vi "SS2 Live_Settings Window.vi"() -> ()   [LabVIEW 2019]
uses:
  SS2 DAQ Parameters 2.ctl
  SS2 Gate Definition.ctl
  SS2 Live_File Information.ctl
  SS2 Live_Gate Characteristics.ctl
  SS2 Live_Image ROI Information.ctl
  Phasor/Image Binning Options.ctl
  SS2 Live_Settings Event.ctl
  SS2 Live_Settings Window Messages.ctl
  SS2 Live_Settings Q Action.ctl
  SS2 Live_Gate Configuration Action.ctl
  SS2 Live_Settings Q Element.ctl
  SS2 Gate Configuration.ctl
  SS2 Live_Globals.vi
  Variant/Variant to Data/Variant to Data.lvlib
panel:
  in  "Tab Control":T1(tab)
  in  "Bitfile Version":string
  in  "Bitfile Path":path
  in  "Buffer Size (# Gates)":u32=1 min=1
  out "Gate Characteristics":T2
  in  "Preset Configuration":u16(ring) items=["User-defined configuration", "Gate Configuration 1", "Gate Configuration 2", "Gate Configuration 3", "Gate Configuration 4", "Gate Configuration 5", "Gate Configuration 6", "Gate Configuration 7"]
  in  "SS2 DAQ Parameters":T3={"10 bits"=FALSE, "# Exposure Sequences"=1, "# 1-bit Frame per Gate"=255, "Gate Shift"=0, "# Gates per Set"=1, "# Sets"=1, "Laser Period"=0.0, "Gate Offset"=0, "Auto-adjust Gate Offset"=FALSE, "Gate Definition"={"gs_psincdec_0"=0, "gs_psincdec_1"=0, "gs_psincdec_2"=0, "gs_psincdec_3"=0, "gs_no_shift_adj_1"=0, "gs_no_shift_adj_2"=0, "gs_no_shift_adj_3"=0}} {"Laser Period" min=0.0; "# 1-bit Frame per Gate" min=255 max=255; "Gate Definition"."gs_psincdec_3" max=1; "Gate Definition"."gs_psincdec_2" max=1; "Gate Definition"."gs_psincdec_1" max=1; "Gate Definition"."gs_psincdec_0" max=1; "# Sets" min=1; "# Gates per Set" min=1}
  in  "Image Binning Options":T5={"Use Image Binning"=FALSE, "X Bin"=1, "Y Bin"=1} {"Y Bin" min=1; "X Bin" min=1}
  in  "Image ROI Information":T6
  in  "# Datasets in Series":i32=1 min=1
  in  "File Information":T7
  in  "Histogram Bins Number":i32=256 min=1 step=1
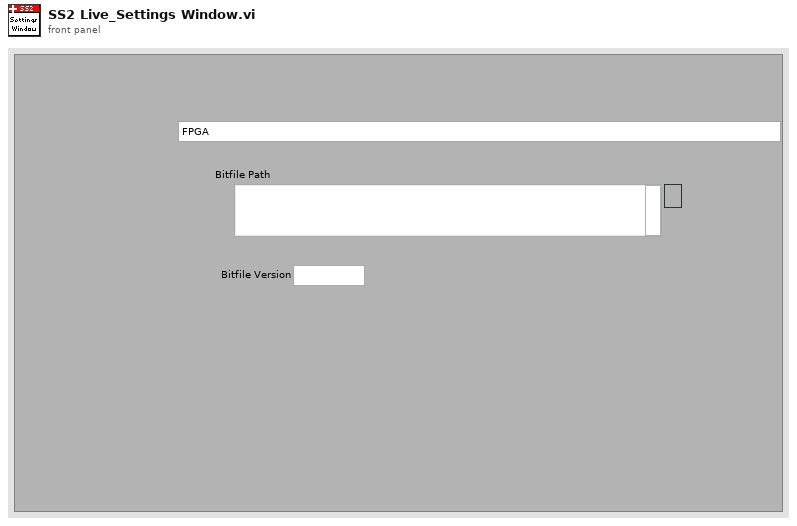
[diagram p1: front panel]
types:
  T1 = enum32{"FPGA", "Acquisition Parameters", "Image Parameters", "File Information", "UI Parameters"}
  T2 = typedef "SS2 Live_Gate Characteristics.ctl" = cluster{"Predicted Gate Width":dbl[unit], "Gate Image Duration":dbl[unit], "Gate Image Exposure":dbl[unit], "Gate Shift":dbl[unit], "Gate Images Span":dbl[unit]}
  T3 = typedef "SS2 DAQ Parameters 2.ctl" = cluster{"10 bits":bool, "# Exposure Sequences":u32, "# 1-bit Frame per Gate":u32, "Gate Shift":u32, "# Gates per Set":u32, "# Sets":u32, "Laser Period":dbl[unit], "Gate Offset":u32, "Auto-adjust Gate Offset":bool, "Gate Definition":T4}
  T4 = typedef "SS2 Gate Definition.ctl" = cluster{"gs_psincdec_0":u32, "gs_psincdec_1":u32, "gs_psincdec_2":u32, "gs_psincdec_3":u32, "gs_no_shift_adj_1":u32, "gs_no_shift_adj_2":u32, "gs_no_shift_adj_3":u32}
  T5 = typedef "Image Binning Options.ctl" = cluster{"Use Image Binning":bool, "X Bin":i32, "Y Bin":i32}
  T6 = typedef "SS2 Live_Image ROI Information.ctl" = cluster{"Save ROI Only":bool, "Left":u16, "Top":u16, "Right":u16, "Bottom":u16, "Use Current ROI":bool}
  T7 = typedef "SS2 Live_File Information.ctl" = cluster{"File Folder":path, "File Name":string, "File Index":u32, "Author":string, "Sample":string, "Compression":bool}
  T8 = typedef "SS2 Live_Settings Q Action.ctl" = enum16{"Idle", "Store Current Configuration", "Rename Current Configuration", "Delete Current Configuration", "Update Image ROI Information", "Quit"}
  T9 = typedef "SS2 Live_Settings Event.ctl" = cluster{"Settings Message":T10, "Sender":string, "Control Label":string, "Data":variant}
  T10 = typedef "SS2 Live_Settings Window Messages.ctl" = enum16{"Idle", "Subscribe", "Unsubscribe", "Refresh Parameter", "Refresh All Parameters", "Quit"}
  T11 = typedef "SS2 Live_Gate Configuration Action.ctl" = enum16{"Get Gate Configuration Name", "Get Configuration by Name", "Add Gate Configuration", "Delete Gate Configuration", "Rename Gate Configuration"}
  T12 = typedef "SS2 Live_Settings Q Element.ctl" = cluster{"Action":T8, "Data":variant}
  T13 = typedef "SS2 Gate Configuration.ctl" = cluster{"Gate Configuration":string, "Gate Offset":u32, "Gate Definition":T4}
  T14 = enum32{"Invalid", "Standard", "Closed", "Hidden", "Minimized", "Maximized"}
  T15 = typedef "SS2 DAQ_Settings Window Messages.ctl" = enum16{"Idle", "Subscribe", "Unsubscribe", "Refresh Parameter", "Refresh All Parameters", "Quit"}
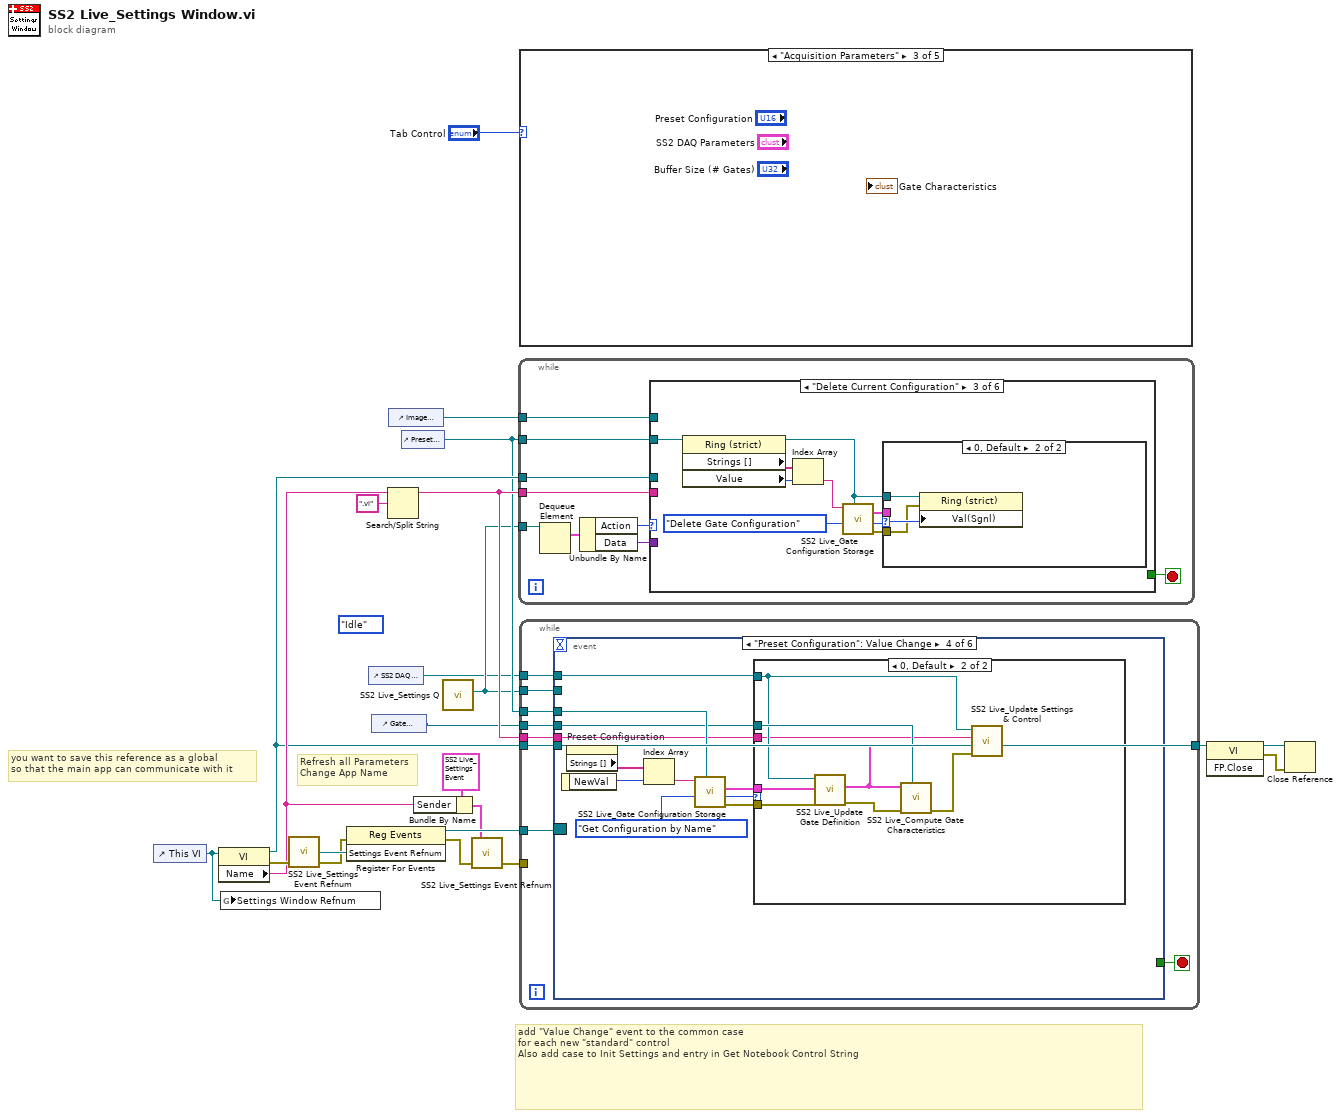
[diagram p0: block diagram]
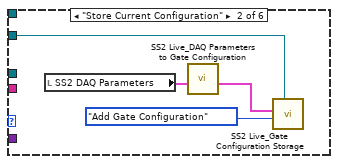
[diagram p3: hidden frame]
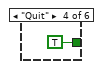
[diagram p5: hidden frame]
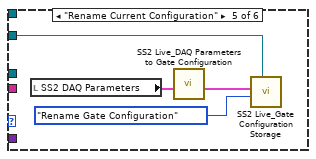
[diagram p6: hidden frame]
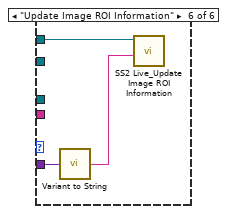
[diagram p7: hidden frame]
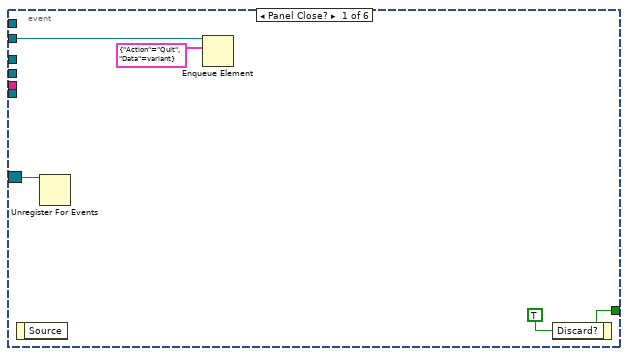
[diagram p8: hidden frame]
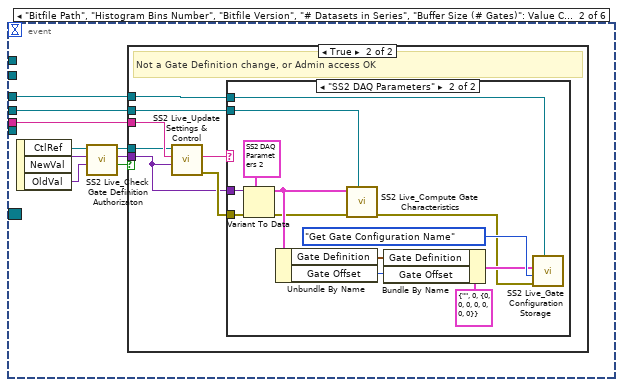
[diagram p9: hidden frame]
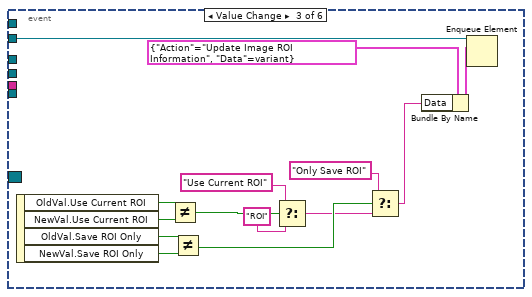
[diagram p12: hidden frame]
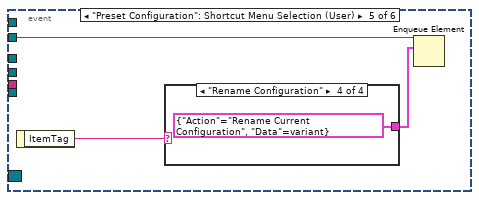
[diagram p14: hidden frame]
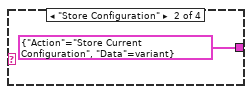
[diagram p16: hidden frame]
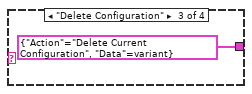
[diagram p17: hidden frame]
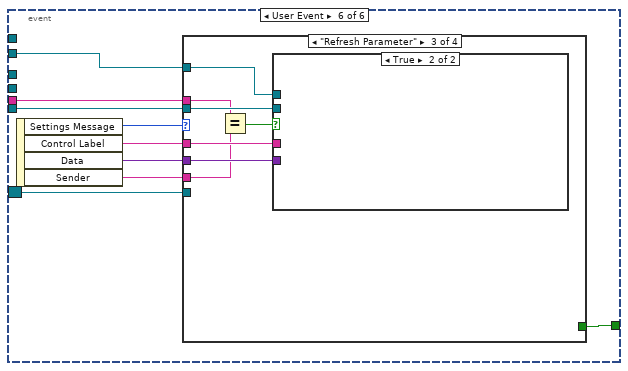
[diagram p18: hidden frame]
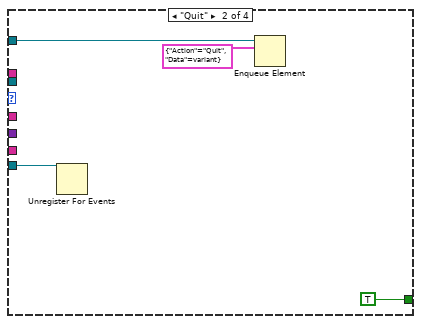
[diagram p20: hidden frame]
diagram:
  (unwired) SS2_Live_Settings_Q_Action."Idle" ("Action")
  # "you want to save this reference as a global\nso that the main app can communicate with it"
  # "add \"Value Change\" event to the common case\nfor each new \"standard\" control\nAlso add case to Init Settings and entry in Get Notebook Control String"
  # "Refresh all Parameters\nChange App Name"
  n1 = control-ref of="This VI"() -> (w6:refnum<vi>)
  n2 = property class="VI"(reference=w6) -> (reference out=w7:refnum<vi>, error out=w16:errorcluster, "Name"=w14:string)  [unwired: 1 in]
  n3 = global write "SS2 Live_Globals.vi" "Settings Window Refnum"(w6) -> ()
  n4 = call "SS2 Live_Settings Event Refnum.vi"("Error In"=w16) -> ("Settings Event Refnum"=w22:refnum<user-event>, "Error Out"=w21:errorcluster)  [unwired: 7 in]
  n5 = register-events(error in=w21, w22) -> (reference out=w19:refnum<event-registration>, error out=w18:errorcluster)  [unwired: 1 in]
  n6 = control-ref of="SS2 DAQ Parameters"() -> (w1:refnum<vi>)
  n7 = control-ref of="Gate Characteristics"() -> (w2:refnum<vi>)
  n8 = Search/Split String(string=w14, search string/char (-)=".vi") -> (substring before match=w9:string)  [unwired: 1 in, 2 out]
  n9 = control-ref of="Image Information"() -> (w4:refnum<vi>)
  n10 = control-ref of="Preset Configuration"() -> (w5:refnum<vi>)
  n11 = Bundle By Name(cluster=T9 {"Settings Message"=enum."Refresh All Parameters", "Sender"="Settings Window", "Control Label"="", "Data"=variant} ("Settings Event"), "Sender"=w14) -> (w15:T9)
  n12 = call "SS2 Live_Settings Q.vi"() -> ("Queue out"=w3:refnum<queue>)  [unwired: 10 in, 1 out]
  n13 = call "SS2 Live_Settings Event Refnum.vi"("Settings Event"=w15, "Error In"=w18) -> ("Error Out"=w12:errorcluster)  [unwired: 6 in, 1 out]
  n14 = while {
    tunnel: w3 -> [w31]
    tunnel: w9 -> [w26]
    tunnel: w7 -> [w25]
    tunnel: w5 -> [w24]
    tunnel: w4 -> [w23]
    stop <- w28 stop-if-true
    n15 = Dequeue Element(queue=w31) -> (element=w30:T12)  [unwired: 2 in, 3 out]
    n16 = Unbundle By Name(w30) -> ("Action"=w29:T8, "Data"=w27:variant)
    n17 = case shown="\"Delete Current Configuration\"" w29 {
      tunnel: [_ _ _ TRUE _ _] -> w28
      tunnel: w27 -> [_ _ _ _ _ w54]
      tunnel: w26 -> [_ _ _ _ _ _]
      tunnel: w25 -> [_ _ _ _ _ _]
      tunnel: w24 -> [_ w32 w43 _ w49 _]
      tunnel: w23 -> [_ _ _ _ _ w55]
      frame "Idle", Default {
      }
      frame "Store Current Configuration" {
        n18 = local read "SS2 DAQ Parameters"() -> (w34:T3)
        n19 = call "SS2 Live_DAQ Parameters to Gate Configuration.vi"("SS2 DAQ Parameters"=w34) -> ("Gate Configuration Definition out"=w33:T13)  [unwired: 10 in]
        n20 = call "SS2 Live_Gate Configuration Storage.vi"("Preset Configuration Refnum"=w32, "Action"=SS2_Live_Gate_Configuration_Action."Add Gate Configuration", "Gate Configuration Definition in"=w33) -> ()  [unwired: 3 in, 6 out]
      }
      frame "Delete Current Configuration" {
        n21 = property class="Ring (strict)"(reference=w43) -> (reference out=w37:refnum<vi>, "Strings []"=w42:string[], "Value"=w41:u16)  [unwired: 1 in, 1 out]
        n22 = Index Array(array=w42, index=w41) -> (element=w40:string)
        n23 = call "SS2 Live_Gate Configuration Storage.vi"("Preset Configuration Refnum"=w37, "Action"=SS2_Live_Gate_Configuration_Action."Delete Gate Configuration", "Gate Configuration Name in"=w40) -> ("Error Out"=w36:errorcluster, "Configuration ID"=w39:i32, "Gate Configuration Definition out"=w38:T13)  [unwired: 3 in, 3 out]
        n24 = case shown="0, Default" w39 {
          selector: w39 -> [_ w47]
          tunnel: w38 -> [_ _]
          tunnel: w37 -> [_ w46]
          tunnel: w36 -> [_ w45]
          frame -1 {
          }
          frame 0, Default {
            n25 = property class="Ring (strict)"(reference=w46, error in=w45, "Val(Sgnl)"=w47) -> ()  [unwired: 2 out]
          }
        }
      }
      frame "Quit" {
      }
      frame "Rename Current Configuration" {
        n26 = local read "SS2 DAQ Parameters"() -> (w51:T3)
        n27 = call "SS2 Live_DAQ Parameters to Gate Configuration.vi"("SS2 DAQ Parameters"=w51) -> ("Gate Configuration Definition out"=w50:T13)  [unwired: 10 in]
        n28 = call "SS2 Live_Gate Configuration Storage.vi"("Preset Configuration Refnum"=w49, "Action"=SS2_Live_Gate_Configuration_Action."Rename Gate Configuration", "Gate Configuration Definition in"=w50) -> ()  [unwired: 3 in, 6 out]
      }
      frame "Update Image ROI Information" {
        n29 = call "Variant to String.vi"("Variant"=w54) -> ("String"=w53:string)  [unwired: 8 in]
        n30 = call "SS2 Live_Update Image ROI Information.vi"("Element Changed"=w53, "Image Information Refnum"=w55) -> ()  [unwired: 8 in, 2 out]
      }
    }
  }
  n31 = case shown="\"Acquisition Parameters\"" "Tab Control" {
    frame "FPGA" {
    }
    frame "UI Parameters" {
    }
    frame "Acquisition Parameters" {
    }
    frame "Image Parameters" {
    }
    frame "File Information" {
    }
  }
  n32 = while {
    tunnel: w7 -> [w61]
    tunnel: [w61] -> w20
    tunnel: w19 -> [w62]
    tunnel: w9 -> [w60]
    tunnel: w12 -> [_]
    tunnel: w3 -> [w59]
    tunnel: w5 -> [w58]
    tunnel: w2 -> [w57]
    tunnel: w1 -> [w56]
    stop <- w63 stop-if-true
    n33 = event shown="[3] \"Preset Configuration\": Value Change" {
      selector: w62 -> [w66 _ _ _ _ w136]
      dyn-events: _ -> [_ _ _ _ _ _]
      timeout: _ -> [_ _ _ _ _ _]
      tunnel: [w67 _ _ _ _ w138] -> w63
      tunnel: w61 -> [_ _ _ _ _ w141]
      tunnel: w60 -> [_ w75 _ w111 _ w139]
      tunnel: w59 -> [w65 _ w110 _ w132 w137]
      tunnel: w58 -> [_ w73 _ w115 _ _]
      tunnel: w57 -> [_ w68 _ w114 _ _]
      tunnel: w56 -> [_ _ _ w113 _ _]
      event Panel Close? {
        w67 = TRUE ("Discard?")
        n34 = event-data() -> ()  [unwired: 1 in, 1 out]
        n35 = Unregister For Events(event registration refnum=w66) -> ()  [unwired: 1 in, 1 out]
        n36 = Enqueue Element(queue=w65, element=T12 {"Action"=enum."Quit", "Data"=variant}) -> ()  [unwired: 2 in, 3 out]
        n37 = event-data("Discard?"=w67) -> ()  [unwired: 1 in, 1 out]
      }
      event "Bitfile Path", "Histogram Bins Number", "Bitfile Version", "# Datasets in Series", "Buffer Size (# Gates)": Value Change {
        n38 = event-data() -> ("CtlRef"=w76:refnum<vi>, "NewVal"=w74:variant, "OldVal"=w70:variant)  [unwired: 1 in]
        n39 = call "SS2 Live_Check Gate Definition Authorizaton.vi"("OldVal"=w70, "NewVal"=w74, "Control Refnum"=w76) -> ("Change Accepted?"=w69:bool, "NewVal"=w71:variant, "Control Refnum"=w72:refnum<vi>)  [unwired: 5 in, 1 out]
        n40 = case shown="True" w69 {
          tunnel: w75 -> [_ w83]
          tunnel: w73 -> [_ w80]
          tunnel: w72 -> [_ w79]
          tunnel: w71 -> [_ w78]
          tunnel: w68 -> [_ w77]
          frame False {
            # "Not admin & Gate Definition change cancelled"
          }
          frame True {
            # "Not a Gate Definition change, or Admin access OK"
            n41 = call "SS2 Live_Update Settings & Control.vi"("Value"=w78, "Sender"=w83, "CtlRef"=w79) -> ("Error Out"=w81:errorcluster, "Control Label"=w82:string)  [unwired: 7 in]
            n42 = case shown="\"SS2 DAQ Parameters\"" w82 {
              tunnel: w78 -> [_ w96]
              tunnel: w81 -> [_ w95]
              tunnel: w80 -> [_ w88]
              tunnel: w77 -> [_ w84]
              frame "", Default {
              }
              frame "SS2 DAQ Parameters" {
                n43 = Variant To Data(error in=w95, type=T3 {"10 bits"=FALSE, "# Exposure Sequences"=0, "# 1-bit Frame per Gate"=255, "Gate Shift"=0, "# Gates per Set"=0, "# Sets"=1, "Laser Period"=0.0, "Gate Offset"=0, "Auto-adjust Gate Offset"=FALSE, "Gate Definition"={"gs_psincdec_0"=0, "gs_psincdec_1"=0, "gs_psincdec_2"=0, "gs_psincdec_3"=0, "gs_no_shift_adj_1"=0, "gs_no_shift_adj_2"=0, "gs_no_shift_adj_3"=0}} ("SS2 DAQ Parameters"), Variant=w96) -> (data=w87:T3, error out=w86:errorcluster)
                n44 = Unbundle By Name(w87) -> ("Gate Definition"=w90:T4, "Gate Offset"=w89:u32)
                n45 = call "SS2 Live_Compute Gate Characteristics.vi"("Gate Characteristics Refnum"=w84, "Error In"=w86, "SS2 DAQ Parameters"=w87) -> ("Error Out"=w85:errorcluster)  [unwired: 7 in, 1 out]
                n46 = Bundle By Name(cluster=T13 {"Gate Configuration"="", "Gate Offset"=0, "Gate Definition"={"gs_psincdec_0"=0, "gs_psincdec_1"=0, "gs_psincdec_2"=0, "gs_psincdec_3"=0, "gs_no_shift_adj_1"=0, "gs_no_shift_adj_2"=0, "gs_no_shift_adj_3"=0}} ("Gate Configuration Definition in"), "Gate Definition"=w90, "Gate Offset"=w89) -> (w91:T13)
                n47 = call "SS2 Live_Gate Configuration Storage.vi"("Preset Configuration Refnum"=w88, "Error In"=w85, "Action"=SS2_Live_Gate_Configuration_Action."Get Gate Configuration Name", "Gate Configuration Definition in"=w91) -> ()  [unwired: 2 in, 6 out]
              }
            }
          }
        }
      }
      event Value Change {
        n48 = event-data() -> ("OldVal.Use Current ROI"=w107:bool, "NewVal.Use Current ROI"=w106:bool, "OldVal.Save ROI Only"=w103:bool, "NewVal.Save ROI Only"=w102:bool)  [unwired: 1 in]
        n49 = Not Equal?(x=w107, y=w106) -> (x != y?=w105:bool)
        n50 = Not Equal?(x=w103, y=w102) -> (x != y?=w100:bool)
        n51 = Select(t="Use Current ROI" ("name (unnamed)"), s=w105, f="ROI" ("name (unnamed)")) -> (s? t:f=w99:string)
        n52 = Select(t="Only Save ROI" ("name (unnamed)"), s=w100, f=w99) -> (s? t:f=w97:string)
        n53 = Bundle By Name(cluster=T12 {"Action"=enum."Update Image ROI Information", "Data"=variant} ("element"), "Data"=w97) -> (w108:T12)
        n54 = Enqueue Element(queue=w110, element=w108) -> ()  [unwired: 2 in, 3 out]
      }
      event "Preset Configuration": Value Change {
        n55 = event-data() -> ("NewVal"=w120:u16)  [unwired: 1 in]
        n56 = property on="Preset Configuration" class="Ring (strict)"() -> ("Strings []"=w121:string[])  [unwired: 2 in, 2 out]
        n57 = Index Array(array=w121, index=w120) -> (element=w119:string)
        n58 = call "SS2 Live_Gate Configuration Storage.vi"("Preset Configuration Refnum"=w115, "Action"=SS2_Live_Gate_Configuration_Action."Get Configuration by Name", "Gate Configuration Name in"=w119) -> ("Error Out"=w112:errorcluster, "Configuration ID"=w117:i32, "Gate Configuration Definition out"=w118:T13)  [unwired: 3 in, 3 out]
        n59 = case shown="0, Default" w117 {
          tunnel: w118 -> [_ w128]
          tunnel: w114 -> [_ w129]
          tunnel: w113 -> [_ w124]
          tunnel: w112 -> [_ w127]
          tunnel: w111 -> [_ w123]
          frame -1 {
          }
          frame 0, Default {
            n60 = call "SS2 Live_Update Gate Definition.vi"("error in (no error)"=w127, "Gate Configuration Definition"=w128, "SS2 DAQ Parameters Refnum"=w124) -> ("error out"=w126:errorcluster, "SS2 DAQ Parameters"=w122:T3)  [unwired: 7 in]
            n61 = call "SS2 Live_Compute Gate Characteristics.vi"("Gate Characteristics Refnum"=w129, "Error In"=w126, "SS2 DAQ Parameters"=w122) -> ("Error Out"=w125:errorcluster)  [unwired: 7 in, 1 out]
            n62 = call "SS2 Live_Update Settings & Control.vi"("Error In"=w125, "Value"=w122, "Sender"=w123, "CtlRef"=w124) -> ()  [unwired: 6 in, 2 out]
          }
        }
      }
      event "Preset Configuration": Shortcut Menu Selection (User) {
        n63 = event-data() -> ("ItemTag"=w131:string)  [unwired: 1 in]
        n64 = case shown="\"Rename Configuration\"" w131 {
          tunnel: [_ T12 {"Action"=enum."Store Current Configuration", "Data"=variant} ("element") T12 {"Action"=enum."Delete Current Configuration", "Data"=variant} ("element") T12 {"Action"=enum."Rename Current Configuration", "Data"=variant} ("element")] -> w130
          frame "", Default {
          }
          frame "Store Configuration" {
          }
          frame "Delete Configuration" {
          }
          frame "Rename Configuration" {
          }
        }
        n65 = Enqueue Element(queue=w132, element=w130) -> ()  [unwired: 2 in, 3 out]
      }
      event User Event {
        n66 = event-data() -> ("Settings Message"=w144:T15, "Control Label"=w143:string, "Data"=w142:variant, "Sender"=w140:string)  [unwired: 1 in]
        n67 = case shown="\"Refresh Parameter\"" w144 {
          tunnel: w143 -> [_ _ w153 _]
          tunnel: w142 -> [_ _ w154 _]
          tunnel: w141 -> [_ _ w155 w174]
          tunnel: w140 -> [_ _ w152 w175]
          tunnel: w139 -> [_ _ w151 w176]
          tunnel: [_ TRUE ("Discard?") _ _] -> w138
          tunnel: w137 -> [_ w147 w149 _]
          tunnel: w136 -> [_ w145 _ _]
          frame "Idle", Default {
          }
          frame "Quit" {
            n68 = Unregister For Events(event registration refnum=w145) -> ()  [unwired: 1 in, 1 out]
            n69 = Enqueue Element(queue=w147, element=T12 {"Action"=enum."Quit", "Data"=variant}) -> ()  [unwired: 2 in, 3 out]
          }
          frame "Refresh Parameter" {
            n70 = Equal?(x=w152, y=w151) -> (x = y?=w150:bool)
            n71 = case shown="True" w150 {
              tunnel: w155 -> [w159 _]
              tunnel: w154 -> [w157 _]
              tunnel: w153 -> [w158 _]
              tunnel: w149 -> [w156 _]
              frame False {
                n72 = case shown="\"Image Information\"" w158 {
                  selector: w158 -> [_ w165]
                  tunnel: w159 -> [_ w166]
                  tunnel: w157 -> [_ w164]
                  tunnel: w156 -> [w163 _]
                  frame "Image Information" {
                    n73 = Bundle By Name(cluster=T12 {"Action"=enum."Update Image ROI Information", "Data"=variant} ("element"), "Data"="Use Current ROI") -> (w161:T12)
                    n74 = Enqueue Element(queue=w163, element=w161) -> ()  [unwired: 2 in, 3 out]
                  }
                  frame "", Default {
                    n75 = call "SS2 Live_Refresh Single Parameter.vi"("Data"=w164, "Control Label"=w165, "VI Ref in"=w166) -> ()  [unwired: 8 in, 1 out]
                  }
                }
              }
              frame True {
              }
            }
          }
          frame "Refresh All Parameters" {
            n76 = First Call?() -> (First Call?: T/F=w172:bool)
            n77 = Not(x=w172) -> (.not. x?=w171:bool)
            n78 = call "SS2 Live_Refresh All Parameters.vi"("Verbose (T)"=w171, "VI Refnum in"=w174) -> ("Error Out"=w167:errorcluster)  [unwired: 9 in]
            n79 = call "Clear Error.vi"("Error In"=w167) -> ("no Error Out"=w168:errorcluster)  [unwired: 8 in]
            n80 = Equal?(x=w176, y=w175) -> (x = y?=w173:bool)
            n81 = property on="Gate Definition" class="Clust (strict)"(error in=w168) -> (error out=w170:errorcluster, "Value"=w169:T4)  [unwired: 1 in, 1 out]
            n82 = case shown="True" w173 {
              tunnel: w174 -> [_ w178]
              frame False {
              }
              frame True {
                n83 = property class="VI"(reference=w178, "FP.State"=T14."Standard" ("State")) -> ()  [unwired: 1 in, 2 out]
              }
            }
            n84 = property on="Gate Definition" class="Clust (strict)"(error in=w170, "Val(Sgnl)"=w169) -> ()  [unwired: 1 in, 2 out]
          }
        }
      }
    }
  }
  n85 = invoke class="VI" method="FP.Close"(reference=w20) -> (reference out=w11:refnum<vi>, error out=w10:errorcluster)  [unwired: 2 in, 1 out]
  n86 = Close Reference(reference=w11, error in (no error)=w10) -> ()  [unwired: 1 out]
